vi "Set Active Item.vi"(8 "error in (no error)":errorcluster, 11 "Data Cluster":T1) -> (0 "error out":errorcluster, 3 "Module Data":T1)   [LabVIEW 2020, in "Peek Window.lvlib"]
uses:
  Peek Window.lvlib
  MHL Data Cluster.ctl
  VI Types/Standard VI Type/Standard VI Type.lvclass
  VI Types/Standard VI Type/Standard VI Type.lvclass/Standard VI Type.ctl
  VI Types/Standard VI Type/Read Full Qualified Name.vi
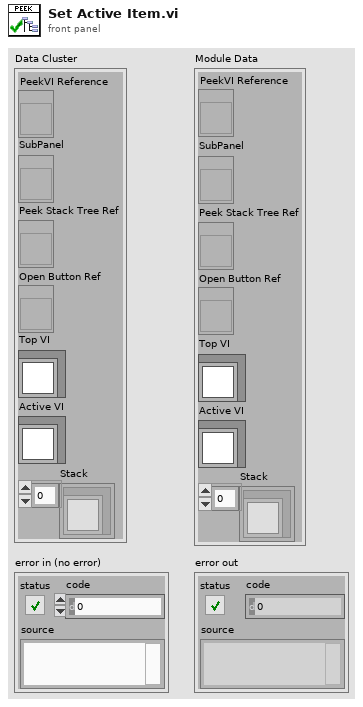
[diagram p1: front panel]
types:
  T1 = typedef "Peek Window.lvlib/MHL Data Cluster.ctl" = cluster{"PeekVI Reference":refnum<vi>, "SubPanel":refnum<vi>, "Peek Stack Tree Ref":refnum<vi>, "Open Button Ref":refnum<vi>, "Top VI":refnum<class "Standard VI Type.lvclass">, "Active VI":refnum<class "Standard VI Type.lvclass">, "Stack":refnum<class "Standard VI Type.lvclass">[]}
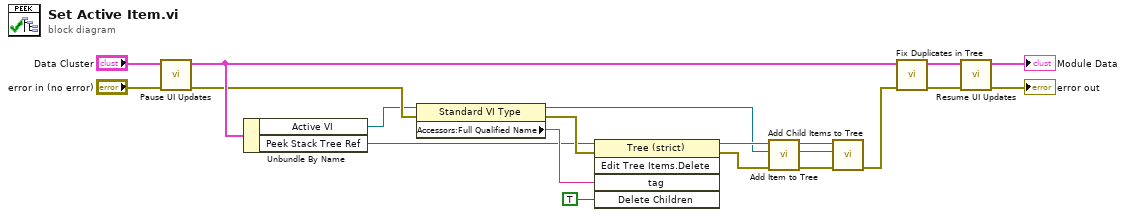
[diagram p0: block diagram]
diagram:
  n1 = call "Pause UI Updates.vi"("error in"="error in (no error)", "Module Data"="Data Cluster") -> ("error out"=w4:errorcluster, "Module Data"=w10:T1)  [unwired: 8 in]
  n2 = Unbundle By Name(w10) -> ("Active VI"=w2:refnum<class "Standard VI Type.lvclass">, "Peek Stack Tree Ref"=w6:refnum<vi>)
  n3 = property class="Standard VI Type"(reference=w2, error in=w4) -> (reference out=w1:refnum<class "Standard VI Type.lvclass">, error out=w7:errorcluster, "Accessors:Full Qualified Name"=w8:string)
  n4 = invoke class="Tree (strict)" method="Edit Tree Items.Delete"(reference=w6, error in=w7, "tag"=w8, "Delete Children"=TRUE) -> (reference out=w5:refnum<vi>, error out=w3:errorcluster)  [unwired: 1 in, 3 out]
  n5 = call-dynamic "Add Item to Tree.vi"("error in (no error)"=w3, "Standard VI Type in"=w1, "Tree Ref in"=w5) -> ("error out"=w11:errorcluster, "Standard VI Type out"=w12:refnum<class "Standard VI Type.lvclass">, "Tree Ref out"=w13:refnum<vi>)  [unwired: 5 in, 1 out]
  n6 = call-dynamic "Add Child Items to Tree.vi"("error in (no error)"=w11, "Standard VI Type in"=w12, "Tree Ref in"=w13) -> ("error out"=w15:errorcluster)  [unwired: 6 in, 2 out]
  n7 = call "Fix Duplicates in Tree.vi"("error in (no error)"=w15, "Data in"=w10) -> ("error out"=w14:errorcluster, "Data out"=w16:T1)  [unwired: 8 in]
  n8 = call "Resume UI Updates.vi"("error in"=w14, "Module Data"=w16) -> ("error out"=→"error out":errorcluster, "Module Data"=→"Module Data":T1)  [unwired: 8 in]
